vi "TPM RSA Encryption Example.vi"() -> ()   [LabVIEW 2021]
uses:
  Key Management/CNG Key Info.ctl
  Key Management/CNG Provider Type.ctl
  Asymmetric Encryption/RSA/RSAEncryptionPadding.ctl
  Key Management/dotNET Crypto Key Management.lvlib
  Asymmetric Encryption/dotNET Crypto Asymmetric Encryption.lvlib
  Utility/dotNET Crypto Utility.lvlib
panel:
  out "error out":errorcluster
  out "Decrypted Data":string
  out "Encrypted Data":string
  out "Key Information":T1
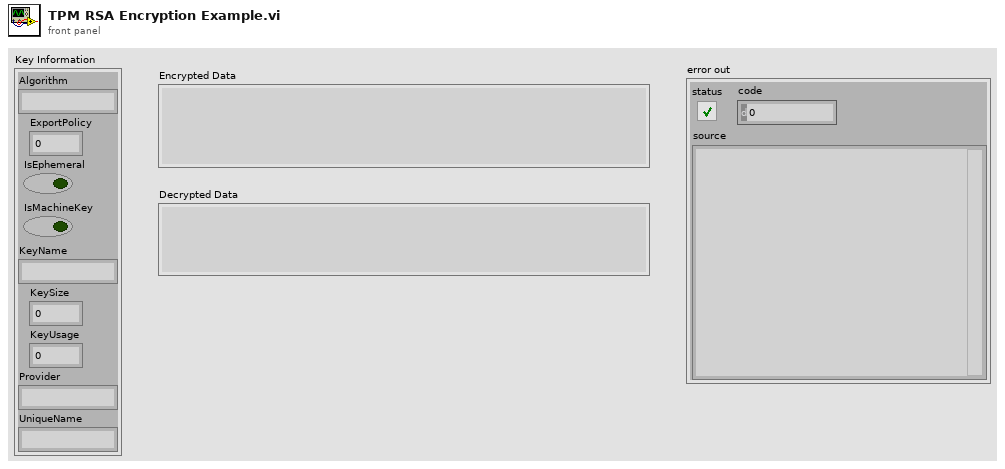
[diagram p1: front panel]
types:
  T1 = typedef "dotNET Crypto Key Management.lvlib/CNG Key Info.ctl" = cluster{"Algorithm":string, "ExportPolicy":i32, "IsEphemeral":bool, "IsMachineKey":bool, "KeyName":string, "KeySize":i32, "KeyUsage":i32, "Provider":string, "UniqueName":string}
  T2 = typedef "dotNET Crypto Asymmetric Encryption.lvlib/RSAEncryptionPadding.ctl" = enum16{"OaepSHA1", "OaepSHA256", "OaepSHA384", "OaepSHA512", "Pkcs1"}
  T3 = typedef "dotNET Crypto Key Management.lvlib/CNG Provider Type.ctl" = enum16{"Microsoft Software Key Storage Provider", "Microsoft Platform Crypto Provider"}
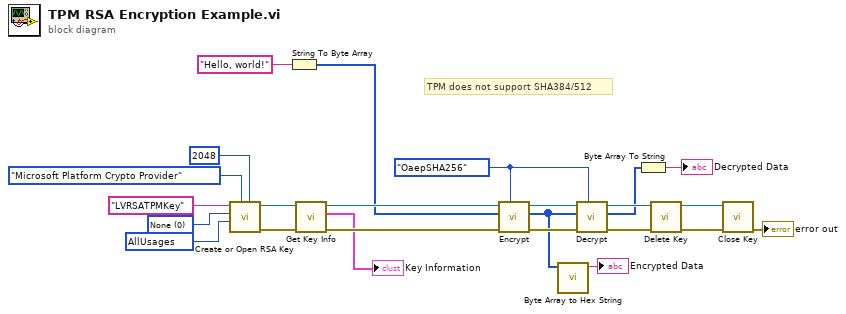
[diagram p0: block diagram]
diagram:
  w3 = 16777215 items=["None"=0, "Decryption"=1, "Signing"=2, "KeyAgreement"=4, "AllUsages"=16777215] ("Key Usage (all usages)")
  w4 = 0 items=["None"=0, "AllowExport"=1, "AllowPlaintextExport"=2, "AllowArchiving"=4, "AllowPlaintextArchiving"=8] ("Export Policy (allow export)")
  w13 = RSAEncryptionPadding."OaepSHA256" ("Padding Mode")
  # "TPM does not support SHA384/512"
  n1 = call "Create or Open RSA Key.vi"("Key Length (2048)"=2048, "Crypto Provider"=CNG_Provider_Type."Microsoft Platform Crypto Provider", "Key Usage (all usages)"=w3, "Export Policy (allow export)"=w4, "Key Name"="LVRSATPMKey") -> ("error out"=w24:errorcluster, ".NET Refnum out"=w23:refnum<k24>)  [unwired: 5 in]
  n2 = String To Byte Array(string="Hello, world!") -> (unsigned byte array=w6:u8[])
  n3 = call "Get Key Info.vi"("error in (no error)"=w24, "CngKey in"=w23) -> ("error out"=w16:errorcluster, "Key Information"=→"Key Information":T1, "CngKey out"=w14:refnum<k24>)  [unwired: 7 in]
  n4 = call "Encrypt.vi"("Padding Mode"=w13, "error in (no error)"=w16, "Raw data in"=w6, "CngKey in"=w14) -> ("error out"=w18:errorcluster, "Encrypted data out"=w11:u8[], "CngKey out"=w17:refnum<k24>)  [unwired: 5 in]
  n5 = call "Byte Array to Hex String.vi"("Byte Array"=w11) -> ("Hex String"=→"Encrypted Data":string)  [unwired: 10 in]
  n6 = call "Decrypt.vi"("Padding Mode"=w13, "error in (no error)"=w18, "Encrypted data in"=w11, "CngKey in"=w17) -> ("error out"=w1:errorcluster, "Raw data out"=w9:u8[], "CngKey out"=w15:refnum<k24>)  [unwired: 5 in]
  n7 = Byte Array To String(unsigned byte array=w9) -> (string=→"Decrypted Data":string)
  n8 = call "Delete Key.vi"("error in (no error)"=w1, "CngKey in"=w15) -> ("error out"=w22:errorcluster, "CngKey out"=w21:refnum<k24>)  [unwired: 8 in]
  n9 = call "Close Key.vi"("error in (no error)"=w22, "CngKey in"=w21) -> ("error out"=→"error out":errorcluster)  [unwired: 9 in]
